vi "Grafica seno.vi"() -> ()   [LabVIEW 2020]
panel:
  in  "stop":bool
  out "Waveform Chart":dbl(graph)
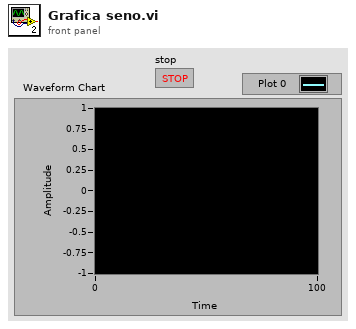
[diagram p1: front panel]
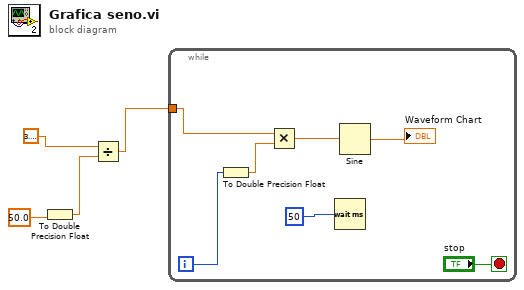
[diagram p0: block diagram]
diagram:
  n1 = To Double Precision Float(number=50.0) -> (double precision float=w2:dbl)
  n2 = Divide(x=3.141592653589793, y=w2) -> (x/y=w4:dbl)
  n3 = while {
    tunnel: w4 -> [w9]
    i -> [w7]
    stop <- "stop" stop-if-true
    n4 = To Double Precision Float(number=w7) -> (double precision float=w8:dbl)
    n5 = Multiply(x=w9, y=w8) -> (x*y=w6:dbl)
    n6 = Wait (ms)(milliseconds to wait=u32 50) -> ()  [unwired: 1 out]
    n7 = Sine(x=w6) -> (sin(x)=→"Waveform Chart":dbl)
  }
